vi "ConvertNormalStringtoHex.vi"(1 "Normal String":string="Hello World!") -> (0 "Hex String":string)   [LabVIEW 2012, in "NFC Driver.lvlib"]
doc: "This VI converts a raw HEX string into it's ASCII representation"
uses:
  NFC Driver.lvlib
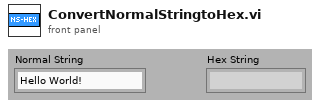
[diagram p1: front panel]
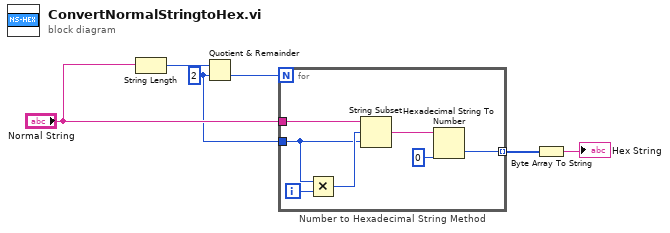
[diagram p0: block diagram]
diagram:
  w2 = u16 2 ("y")
  n1 = String Length(string="Normal String") -> (length=w4:i32)
  n2 = Quotient & Remainder(x=w4, y=w2) -> (floor(x/y)=w1:i32)  [unwired: 1 out]
  n3 = for "Number to Hexadecimal String Method" {
    N: w1 -> [_]
    tunnel: [w8] -> w6 mode=indexing
    tunnel: "Normal String" -> [w13]
    tunnel: w2 -> [w10]
    i -> [w12]
    n4 = Multiply(x=w10, y=w12) -> (x*y=w11:i32)
    n5 = String Subset(string=w13, offset (0)=w11, length (rest)=w10) -> (substring=w9:string)
    n6 = Hexadecimal String To Number(string=w9, default (0uL)=u8 0 ("default (0 U32)")) -> (number=w8:u8)  [unwired: 1 in, 1 out]
  }
  n7 = Byte Array To String(unsigned byte array=w6) -> (string=→"Hex String":string)
